vi "reader.vi"() -> ()   [LabVIEW 2020]
uses:
  <vilib>/addons/Sound and Vibration/svt_Controls/subVIs/Octave Graph.ctl
  <vilib>/addons/_NISVFA/_Shared subVIs/Common/SVL Set dB Reference (1 Ch).vi
  <vilib>/addons/_NISVFA/_Shared subVIs/Common/SVL Set dB Reference (variant).vi
  <vilib>/addons/_NISVFA/_Shared subVIs/Common/svc_Caller VI Returned in Error Source.vi
  <vilib>/addons/Sound and Vibration/svt_Octave_2014 standard/SVT Third-octave Analysis (1 Ch).vi
  <vilib>/addons/Sound and Vibration/svt_Weighting/SVT A, B, C Weighting Filter (Fixed Rates) (1 Ch).vi
  <vilib>/addons/Sound and Vibration/svt_Level/SVL Leq Sound Level (1 Ch).vi
  <vilib>/addons/Sound and Vibration/svt_Weighting/SoundVib_ABCWeighting.lvlib
  <vilib>/addons/Sound and Vibration/svt_Level/SoundVib_SoundLevel.lvlib
  <vilib>/addons/Sound and Vibration/svt_Octave/SoundVib_Octave_2014 standard.lvlib
panel:
  in  "Tab Control":enum32{"Page 1", "Page 2", "Page 3"}(tab)
  out "?":waveform(dbl)(graph)
  out "Peak":dbl
  out "?":dbl
  out "?":dbl
  in  "stop":bool
  in  "weighting":u16(ring) items=["Linear", "A-weighting", "B-weighting", "C-weighting"]
  in  "Mode":enum16{"Slow", "Fast"}(ring)
  in  "Restart":bool
  in  "restart everaging (F)":bool
  out "Leq sound level [dB EU]":dbl format="%.2f"
  out "Octave graph":T1
  # "dB"
  # "PEAK"
  # "Leq"
  # "MAX"
  # "dB"
  # "MAX"
  # "dB"
  # "MIN"
  # "dB"
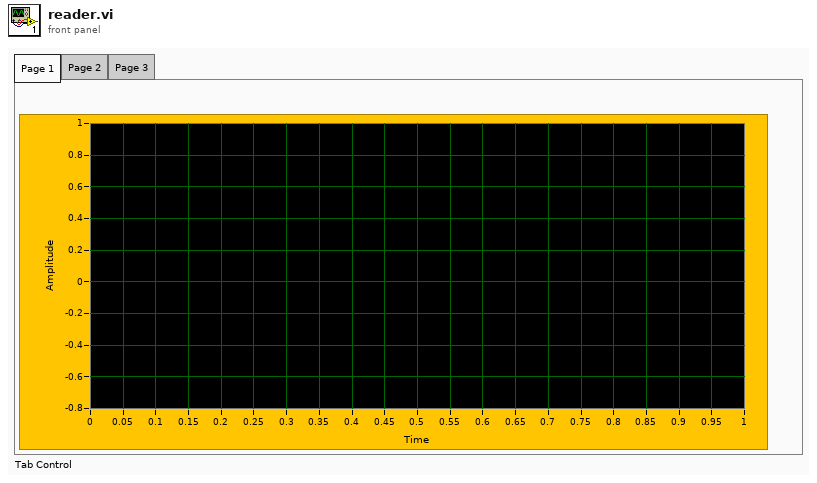
[diagram p1: front panel]
types:
  T1 = typedef "Octave Graph.ctl" = cluster{"nominal frequencies [Hz]":dbl[], "band power [dB EU]":dbl[]}
  T2 = cluster{"nominal frequencies [Hz]":dbl[], "band power":dbl[]}
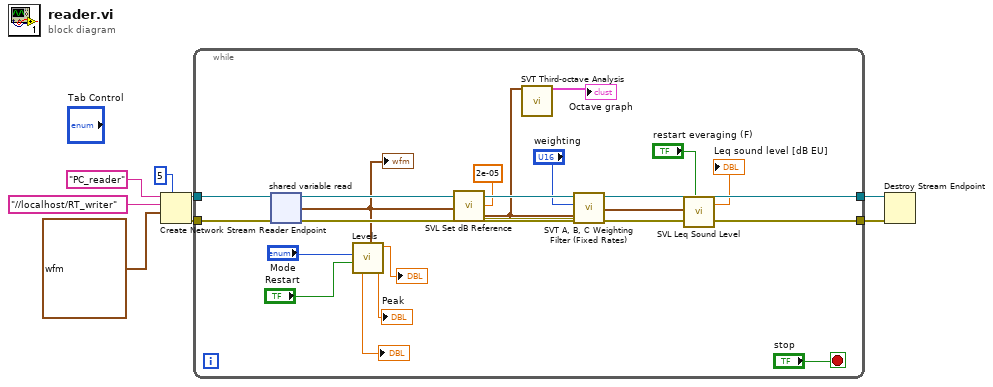
[diagram p0: block diagram]
diagram:
  n1 = Create Network Stream Reader Endpoint(7:5 ("writer buffer size"), 9:waveform(dbl) {"t0"=timestamp(0 s since 1904-01-01), "dt"=1.0, "Y"=[]} ("time signal"), 10:"//localhost/RT_writer" ("writer url"), 11:"PC_reader" ("writer name")) -> (0:w4:errorcluster, 3:w3:refnum<k21>)  [unwired: 3 in]
  n2 = while {
    tunnel: w4 -> [w28]
    tunnel: w3 -> [w27]
    tunnel: [w26] -> w2
    tunnel: [w25] -> w1
    stop <- "stop" stop-if-true
    n3 = shared-variable-read(w27, w28) -> (w26:refnum<k21>, w25:errorcluster, w16:waveform(dbl))  [unwired: 1 in, 1 out]
    "?" <- w16
    n4 = call "Levels.vi"("Restart"="Restart", "Mode"="Mode", "time signal"=w16) -> ("Lmin"=→"?":dbl, "Lpeak"=→"Peak":dbl, "Lmax"=→"?":dbl)  [unwired: 6 in]
    n5 = call-poly <vilib>:"SVL Set dB Reference.vi"("dB reference [EU]"=2e-05, "scaled signal in [EU]"=w16) -> ("error out"=w22:errorcluster, "scaled signal out [EU]"=w11:waveform(dbl))  [unwired: 8 in]
    n6 = call-poly <vilib>:"SVT Third-octave Analysis.vi"("scaled signal [EU]"=w11) -> ("octave spectrum"=→"Octave graph":T2)  [unwired: 9 in, 5 out]
    n7 = call-poly <vilib>:"SVT A, B, C Weighting Filter (Fixed Rates).vi"("error in (no error)"=w22, "weighting"="weighting", "scaled signal [EU]"=w11) -> ("error out"=w20:errorcluster, "weighted signal [EU]"=w21:waveform(dbl))  [unwired: 6 in]
    n8 = call-poly <vilib>:"SVL Leq Sound Level.vi"("restart averaging (F)"="restart everaging (F)", "error in (no error)"=w20, "scaled signal [EU]"=w21) -> ("Leq sound level [dB EU]"=→"Leq sound level [dB EU]":dbl)  [unwired: 6 in, 2 out]
  }
  n9 = Destroy Stream Endpoint(8:w1, 11:w2) -> ()  [unwired: 1 out]
